vi "get_or_set_modifier_values.vi"(5 "modifier index":i32, 6 "clamp output values?":bool[](array[boolean]), 7 "action":T1, 8 "error in (no error)":errorcluster, 10 "modifier values in":dbl[](array[numeric]), 11 "GenericTrajectory in":refnum<class "TrajectoryDL090201FrameScan.lvclass">) -> (0 "error out":errorcluster, 2 "modifier values out":dbl[](array[numeric]), 3 "GenericTrajectory out":refnum<class "TrajectoryDL090201FrameScan.lvclass">)   [LabVIEW 2010, in "TrajectoryDL090201FrameScan.lvclass"]
uses:
  TrajectoryDL090201FrameScan.lvclass
  common/enumerations/functional_global_action_enum.ctl
  TrajectoryDL091126GenericVoxel/TrajectoryDL091126GenericVoxel/TrajectoryDL091126GenericVoxel.lvclass
panel:
  out "Waveform Graph":i16[](graph)
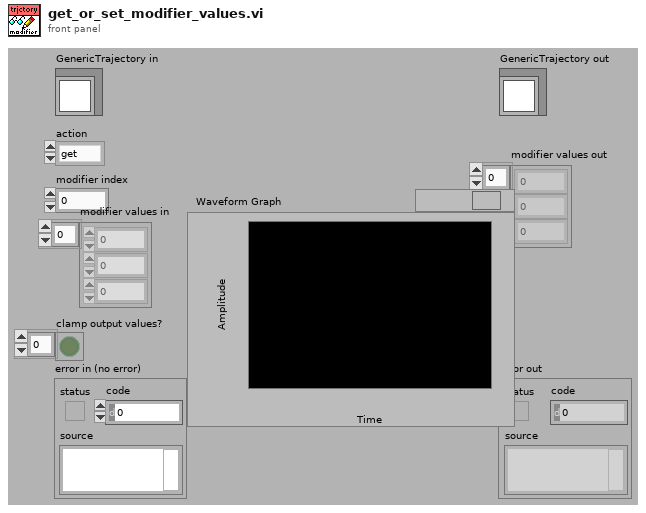
[diagram p1: front panel]
types:
  T1 = typedef "functional_global_action_enum.ctl" = enum16{"get", "set", "reset"}
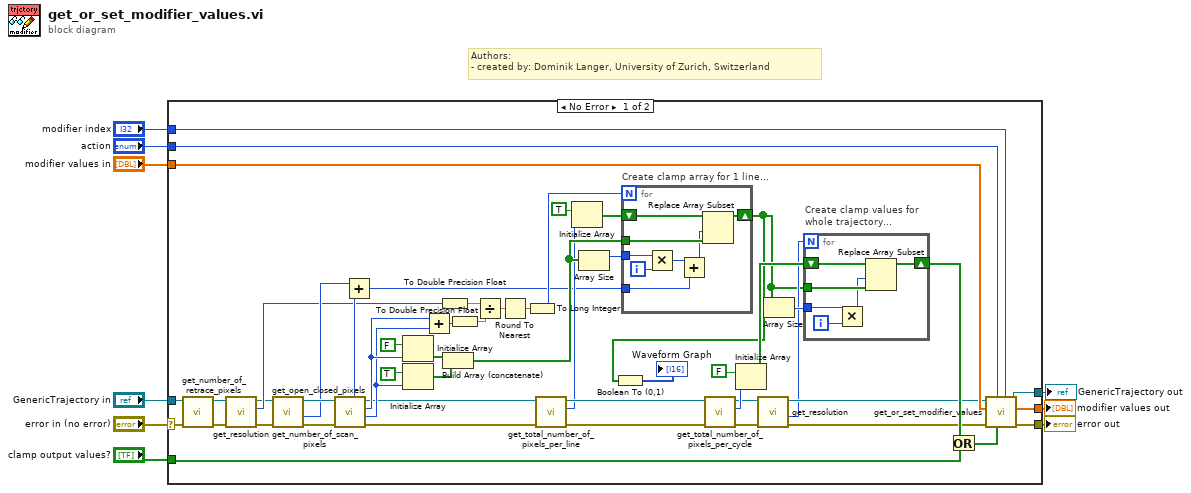
[diagram p0: block diagram]
diagram:
  # "Authors: \n- created by: Dominik Langer, University of Zurich, Switzerland"
  n1 = case shown="No Error" "error in (no error)" {
    selector: "error in (no error)" -> [w51 w79]
    tunnel: [w62 w79] -> w9
    tunnel: [w61 w78] -> w8
    tunnel: "modifier index" -> [w60 _]
    tunnel: "action" -> [w59 _]
    tunnel: "modifier values in" -> [w58 w78]
    tunnel: "GenericTrajectory in" -> [w52 w77]
    tunnel: [w53 w77] -> w2
    tunnel: "clamp output values?" -> [w27 _]
    frame No Error {
      n2 = call "get_number_of_retrace_pixels.vi"("error in (no error)"=w51, "DL090201FrameScanTrajectory in"=w52) -> ("error out"=w11:errorcluster, "DL090201FrameScanTrajectory out"=w13:refnum<class "TrajectoryDL090201FrameScan.lvclass">)  [unwired: 7 in, 1 out]
      n3 = call-dynamic "get_resolution.vi"("error in (no error)"=w11, "TrajectoryDL090201FrameScan in"=w13) -> ("error out"=w10:errorcluster, "x"=w14:i32, "TrajectoryDL090201FrameScan out"=w12:refnum<class "TrajectoryDL090201FrameScan.lvclass">)  [unwired: 6 in, 1 out]
      n4 = call "get_number_of_scan_pixels.vi"("error in (no error)"=w10, "DL090201FrameScanTrajectory in"=w12) -> ("error out"=w25:errorcluster, "number of scan cut-off pixels"=w18:i32, "DL090201FrameScanTrajectory out"=w24:refnum<class "TrajectoryDL090201FrameScan.lvclass">)  [unwired: 6 in, 1 out]
      n5 = call-dynamic "get_open_closed_pixels.vi"("error in (no error)"=w25, "TrajectoryDL090201FrameScan in"=w24) -> ("error out"=w30:errorcluster, "number of closed pixels"=w46:i32, "number of open pixels"=w47:i32, "TrajectoryDL090201FrameScan out"=w29:refnum<class "TrajectoryDL090201FrameScan.lvclass">, "number of offset pixels"=w38:i32)  [unwired: 5 in]
      n6 = Add(x=w18, y=w38) -> (x+y=w32:i32)
      n7 = Initialize Array(FALSE, w47) -> (w55:bool[])
      n8 = Initialize Array(TRUE, w46) -> (w54:bool[])
      n9 = Add(x=w47, y=w46) -> (x+y=w34:i32)
      n10 = To Double Precision Float(number=w14) -> (double precision float=w31:dbl)
      n11 = Build Array (concatenate)(w55, w54) -> (w43:bool[])
      n12 = To Double Precision Float(number=w34) -> (double precision float=w37:dbl)
      n13 = Divide(x=w31, y=w37) -> (x/y=w36:dbl)
      n14 = Round To Nearest(number=w36) -> (nearest integer value=w35:dbl)
      n15 = To Long Integer(number=w35) -> (32bit integer=w33:i32)
      n16 = call-dynamic "get_total_number_of_pixels_per_line.vi"("error in (no error)"=w30, "DL090201FrameScanTrajectory in"=w29) -> ("error out"=w40:errorcluster, "total number of pixels per line"=w39:i32, "DL090201FrameScanTrajectory out"=w41:refnum<class "TrajectoryDL090201FrameScan.lvclass">)  [unwired: 7 in]
      n17 = Initialize Array(TRUE, w39) -> (w17:bool[])
      n18 = Array Size(array=w43) -> (size(s)=w42:i32)
      n19 = for "Create clamp array for 1 line..." {
        N: w33 -> [_]
        tunnel: w43 -> [w69]
        shift-right: [w66] -> w15
        shift-left: w17 -> [w70]
        tunnel: w42 -> [w68]
        tunnel: w32 -> [w63]
        i -> [w67]
        n20 = Multiply(x=w68, y=w67) -> (x*y=w65:i32)
        n21 = Add(x=w65, y=w63) -> (x+y=w64:i32)
        n22 = Replace Array Subset(array=w70, new element=w69, index=w64) -> (w66:bool[])
      }
      n23 = Boolean To (0,1)(Boolean=w15) -> (0, 1=→"Waveform Graph":i16[])
      n24 = call-dynamic "get_total_number_of_pixels_per_cycle.vi"("error in (no error)"=w40, "TrajectoryDL090201FrameScan in"=w41) -> ("error out"=w22:errorcluster, "total number of pixels per cycle"=w49:i32, "TrajectoryDL090201FrameScan out"=w23:refnum<class "TrajectoryDL090201FrameScan.lvclass">)  [unwired: 7 in]
      n25 = Initialize Array(FALSE, w49) -> (w45:bool[])
      n26 = call-dynamic "get_resolution.vi"("error in (no error)"=w22, "TrajectoryDL090201FrameScan in"=w23) -> ("error out"=w21:errorcluster, "y"=w19:i32, "TrajectoryDL090201FrameScan out"=w20:refnum<class "TrajectoryDL090201FrameScan.lvclass">)  [unwired: 6 in, 1 out]
      n27 = Array Size(array=w15) -> (size(s)=w48:i32)
      n28 = for "Create clamp values for whole trajectory..." {
        N: w19 -> [_]
        shift-right: [w74] -> w28
        shift-left: w45 -> [w76]
        tunnel: w15 -> [w75]
        tunnel: w48 -> [w72]
        i -> [w73]
        n29 = Multiply(x=w72, y=w73) -> (x*y=w71:i32)
        n30 = Replace Array Subset(array=w76, new element=w75, index=w71) -> (w74:bool[])
      }
      n31 = Or(x=w27, y=w28) -> (x .or. y?=w26:bool[])
      n32 = call-parent "get_or_set_modifier_values.vi"("modifier index"=w60, "clamp output values?"=w26, "action"=w59, "error in (no error)"=w21, "modifier values in"=w58, "GenericTrajectory in"=w20) -> ("error out"=w62:errorcluster, "modifier values out"=w61:dbl[], "GenericTrajectory out"=w53:refnum<class "TrajectoryDL090201FrameScan.lvclass">)  [unwired: 3 in]
    }
    frame Error {
    }
  }
  "error out" <- w9
  "GenericTrajectory out" <- w2
  "modifier values out" <- w8
